vi "GCM_Interface.vi"() -> ()   [LabVIEW 2014]
uses:
  <vilib>/Utility/miscctls.llb/LVPointTypeDef.ctl
  Utilites/Controls/GCM_Data.ctl
  Framework/_Plugins/GCMPlugin/GCMPlugin.lvclass
  Framework/_Plugins/_EmptyPlugin/_EmptyPlugin.lvclass
  Framework/SelectedPluginStorage/SelectedPluginStorage.lvclass
  Framework/_Plugins/GCMSettingsScreen/GCMSettingsScreen.lvclass
  Utilites/Controls/GCM_State.ctl
  Framework/_Plugins/_LVCMPlugin/GCMPlugin_EventsOut.ctl
  Framework/_Plugins/GCMPlugin/GCMPlugin.lvclass/GCMPlugin.ctl
  <vilib>/Utility/cursorutil.llb/Set Cursor (Icon Pict).vi
  Framework/PluginsThread/PluginsLoaderService/PluginsLoaderService.lvclass
  Framework/PluginsThread/PluginsLoaderCommander/PluginsLoaderCommander.lvclass
panel:
  in  "SettingsButton":bool
  out "Item Type":string="Item type"
  out "Current Item":string="Item name"
  in  "Stay on top?":bool
  in  "Plugins":i32(listbox)
  in  "VeritechLogo":bool
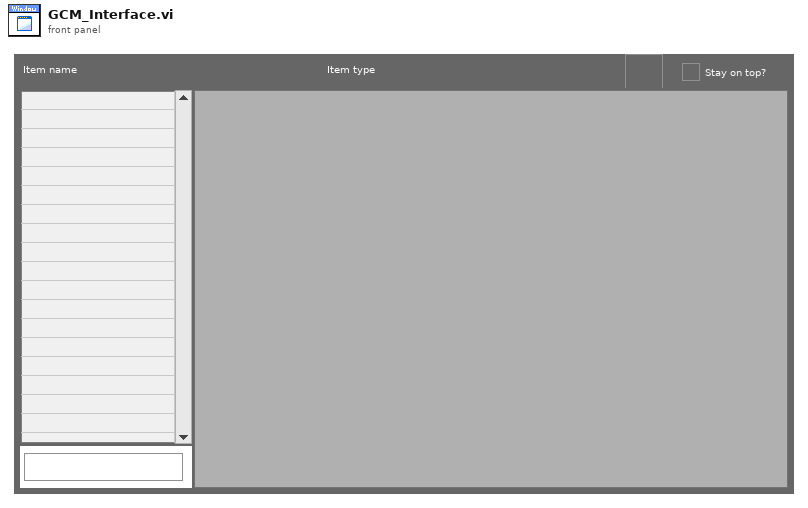
[diagram p1: front panel]
types:
  T1 = typedef "LVPointTypeDef.ctl" = cluster{"Horizontal":i16, "Vertical":i16}
  T2 = typedef "GCMPlugin.lvclass/GCMPlugin_EventsOut.ctl" = cluster{"ItemEdited":refnum<user-event>}
  T3 = typedef "GCM_State.ctl" = enum16{"Initialize", "WaitForEvent", "ShowPluginInterface", "Stop", "LoadDefaultPlugin"}
  T4 = typedef "GCM_Data.ctl" = cluster{"CurrentProjectItem":refnum<vi>, "AvailablePlugins":refnum<class "GCMPlugin.lvclass">[], "EmptyPlugin":refnum<class "_EmptyPlugin.lvclass">, "CurrentPlugin":refnum<class "GCMPlugin.lvclass">, "SelectedPluginStorage":refnum<class "SelectedPluginStorage.lvclass">, "SettingsPlugin":refnum<class "GCMSettingsScreen.lvclass">}
  T5 = enum32{"Invalid", "Default", "Floating", "Floating/Auto-Hide", "Modal"}
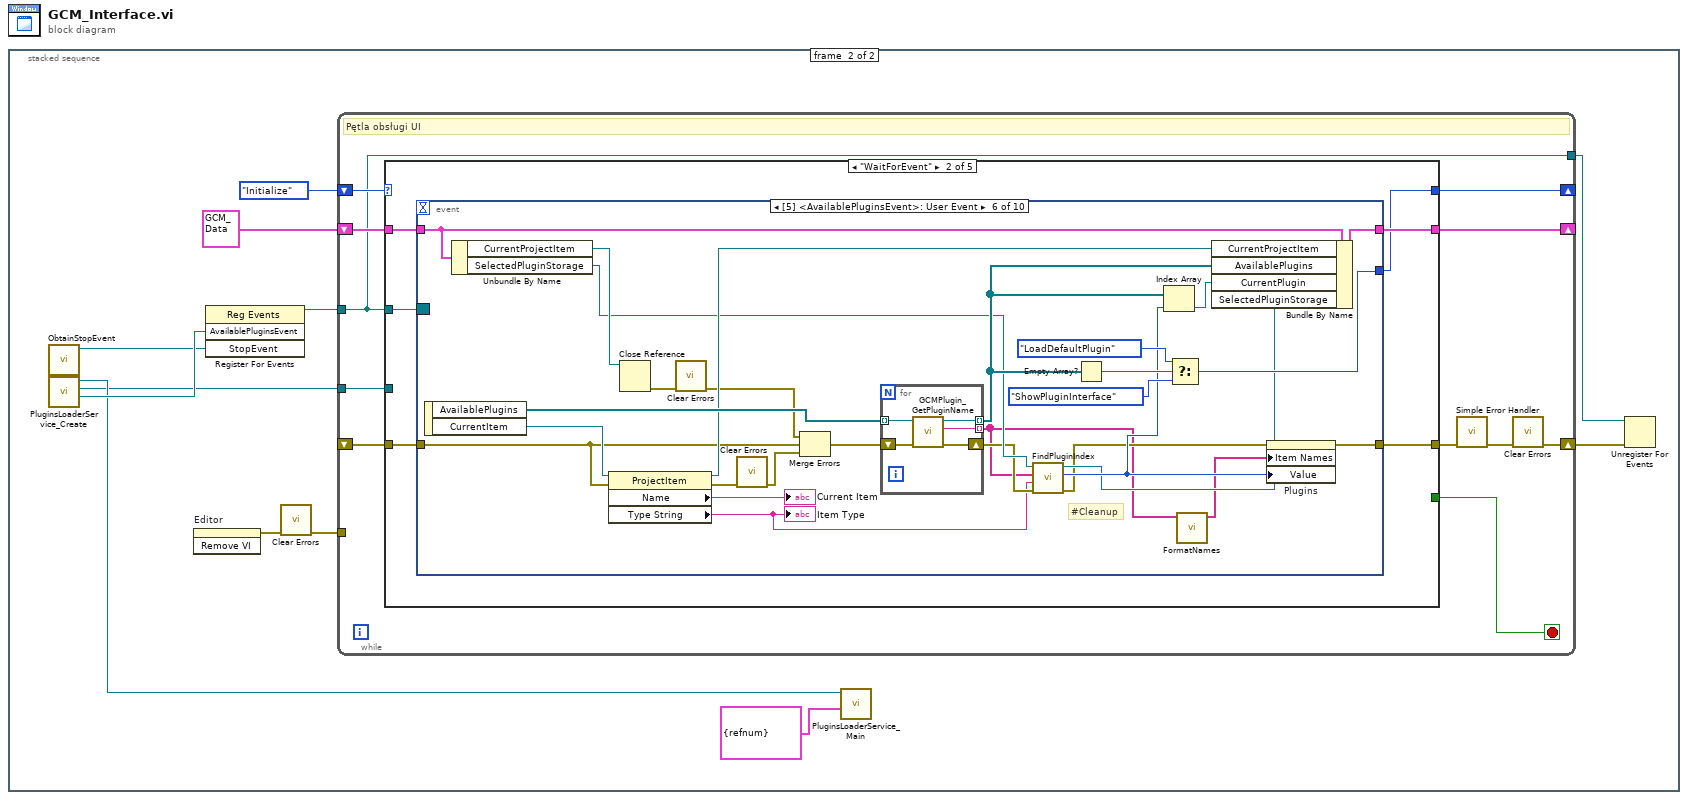
[diagram p0: block diagram]
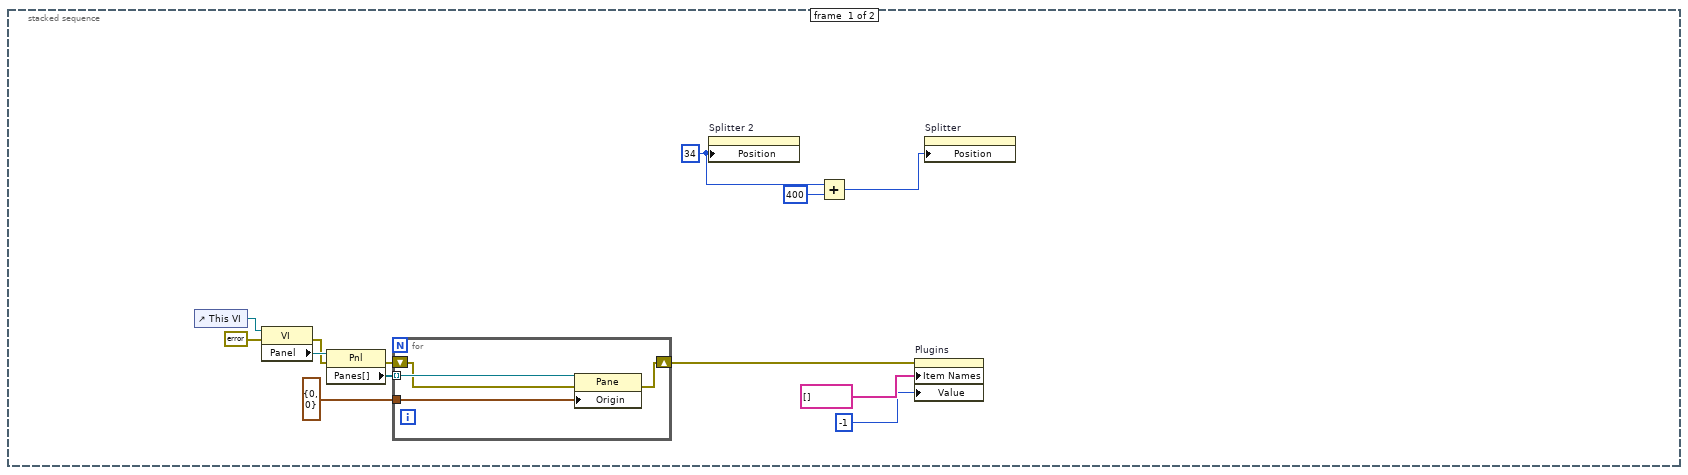
[diagram p2: hidden frame]
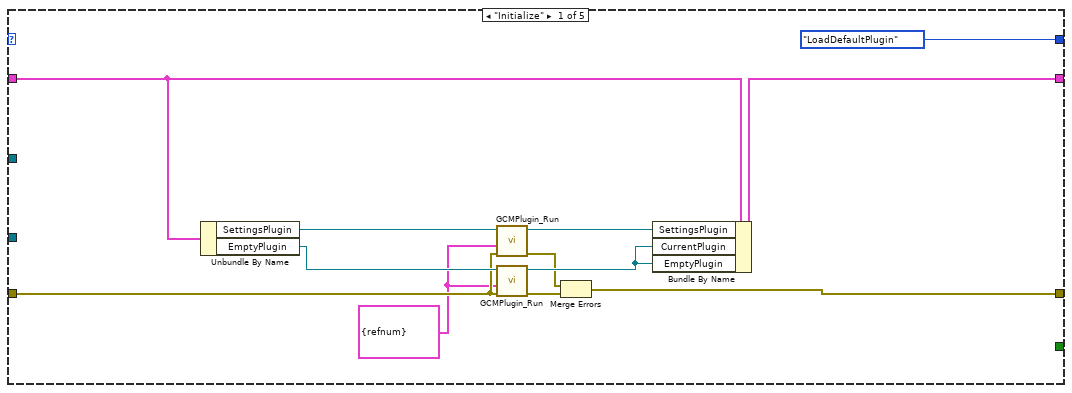
[diagram p3: hidden frame]
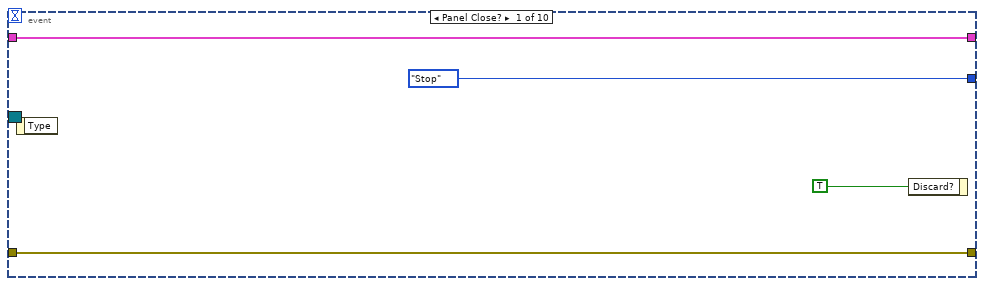
[diagram p4: hidden frame]
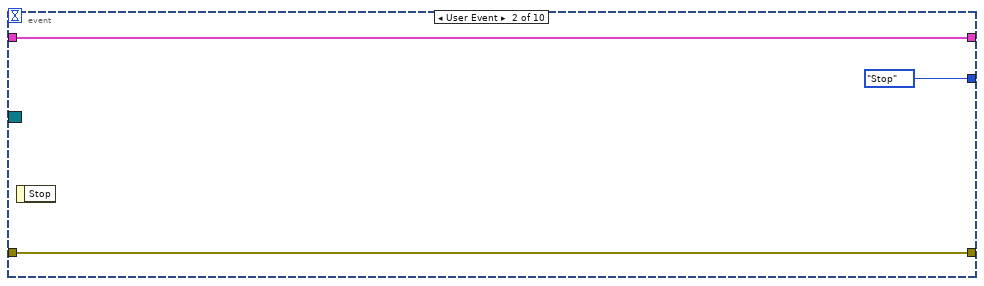
[diagram p5: hidden frame]
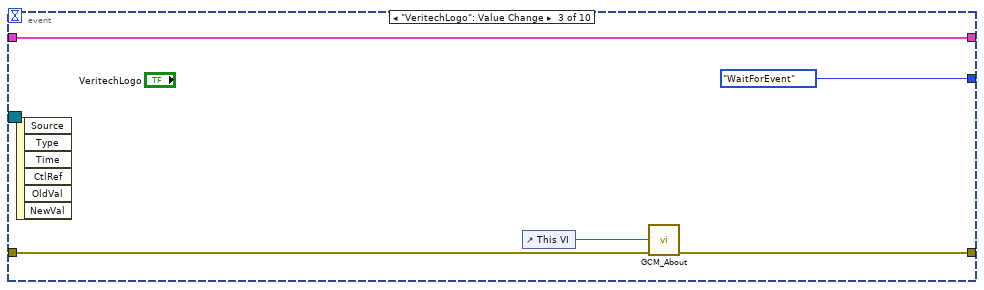
[diagram p6: hidden frame]
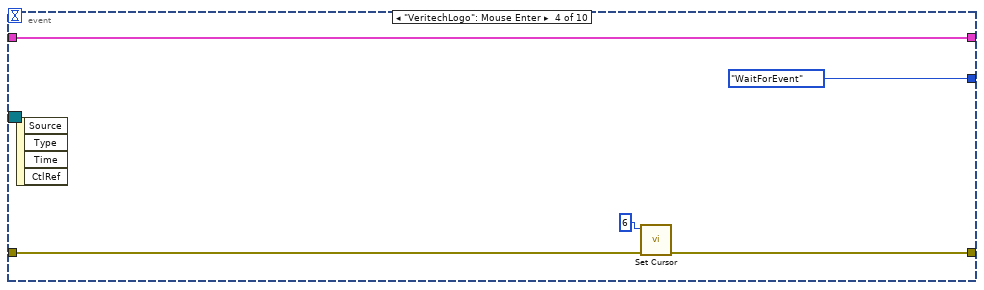
[diagram p7: hidden frame]
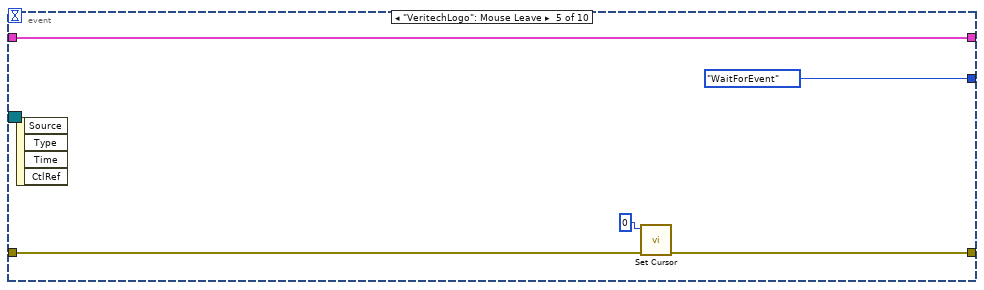
[diagram p8: hidden frame]
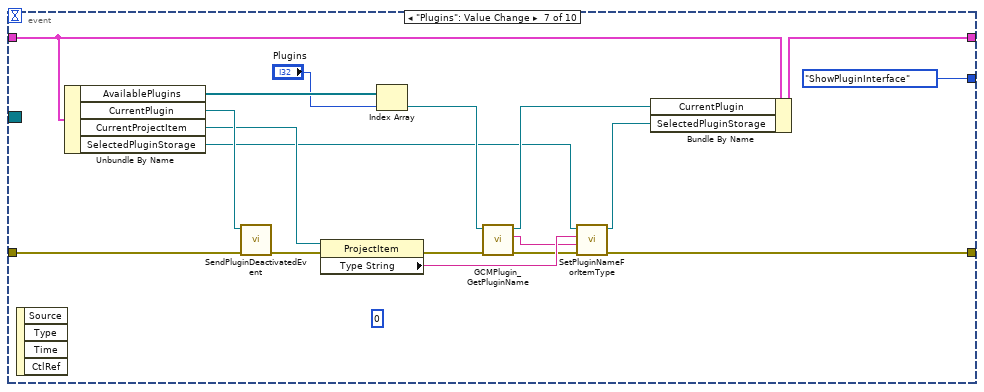
[diagram p9: hidden frame]
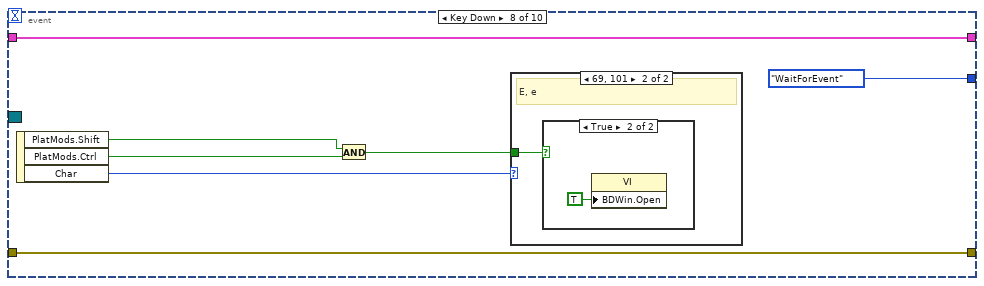
[diagram p10: hidden frame]
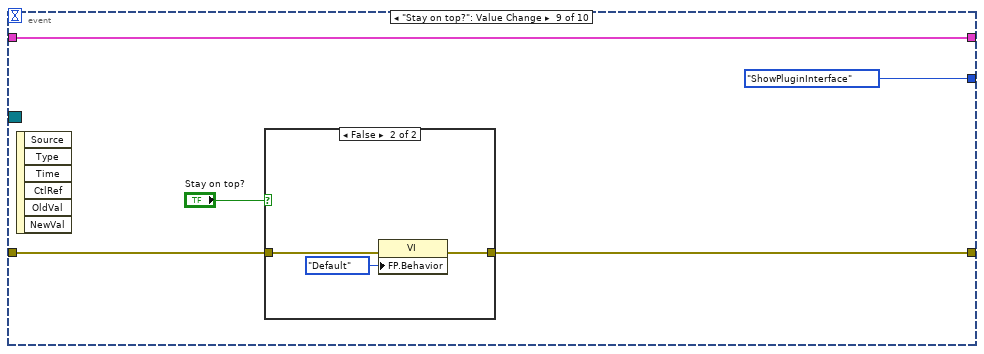
[diagram p13: hidden frame]
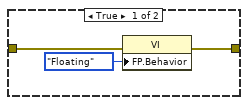
[diagram p14: hidden frame]
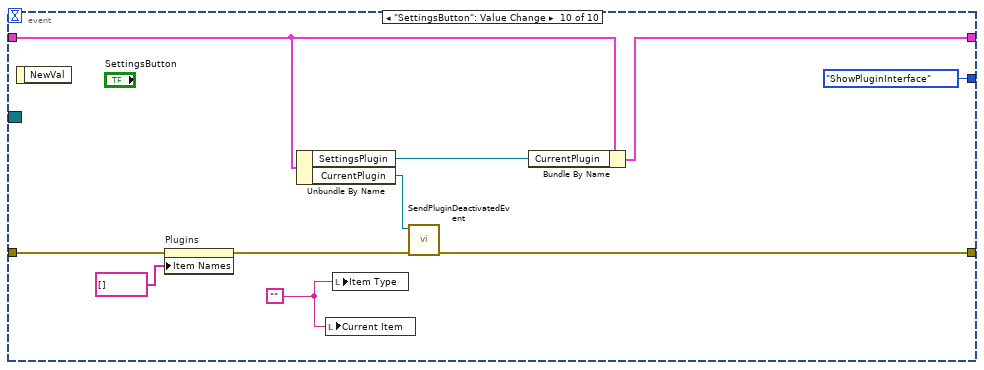
[diagram p15: hidden frame]
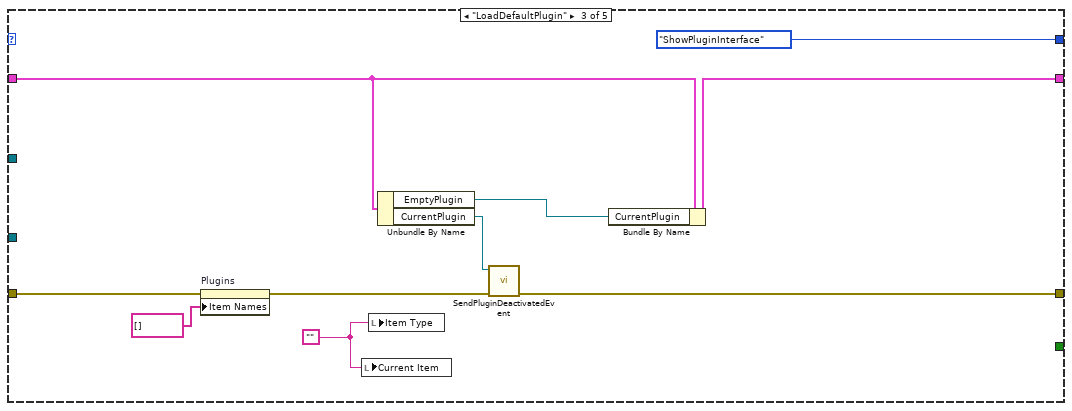
[diagram p16: hidden frame]
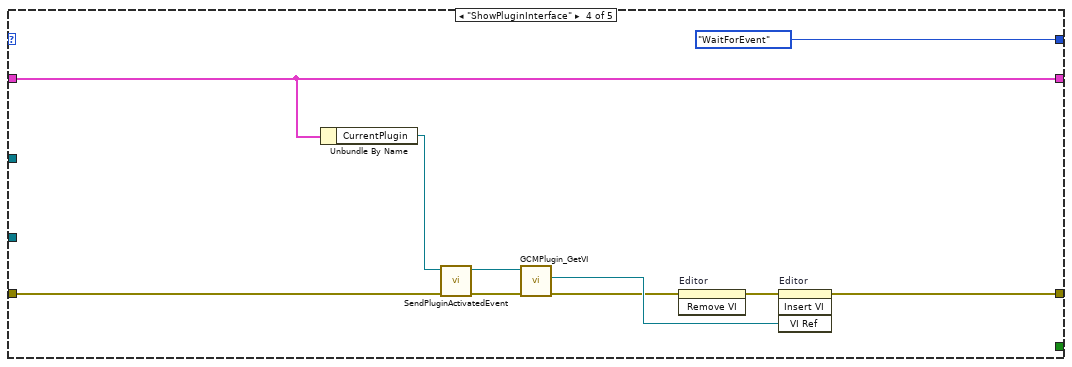
[diagram p17: hidden frame]
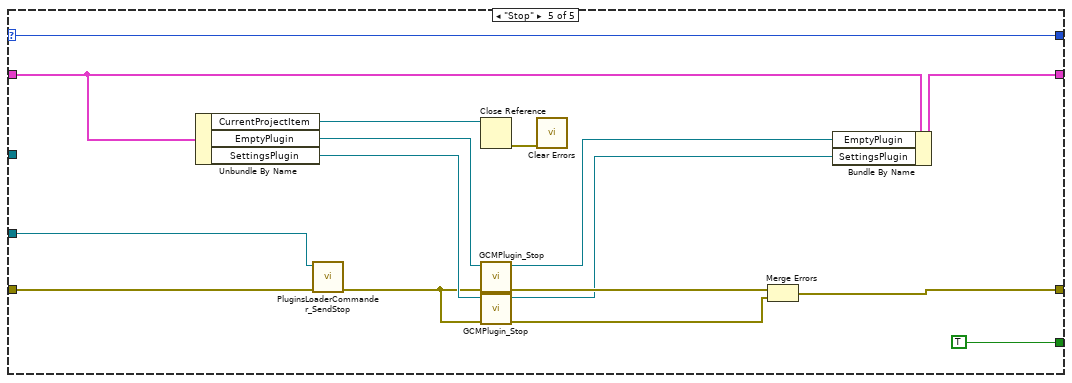
[diagram p18: hidden frame]
diagram:
  n1 = stacked-sequence {
    frame #0 {
      w3 = 34 ("Splitter Position")
      n2 = control-ref of="This VI"() -> (w13:refnum<vi>)
      n3 = property class="VI"(reference=w13, error in=errorcluster {"status"=FALSE, "code"=0, "source"=""} ("error in (no error)")) -> (error out=w11:errorcluster, "Panel"=w12:refnum<vi>)  [unwired: 1 out]
      n4 = property class="Pnl"(reference=w12, error in=w11) -> (error out=w8:errorcluster, "Panes[]"=w9:refnum<vi>[])  [unwired: 1 out]
      n5 = for {
        tunnel: w9 -> [w17] mode=indexing
        shift-right: [w15] -> w6
        shift-left: w8 -> [w16]
        tunnel: T1 {"Horizontal"=0, "Vertical"=0} ("Origin") -> [w14]
        n6 = property class="Pane"(reference=w17, error in=w16, "Origin"=w14) -> (error out=w15:errorcluster)  [unwired: 1 out]
      }
      n7 = property on="Splitter 2" class="Splitter"("Position"=w3) -> ()  [unwired: 2 in, 2 out]
      n8 = Add(x=w3, y=400) -> (x+y=w1:i32)
      n9 = property on="Plugins" class="LstBox (strict)"(error in=w6, "Item Names"=string[] [], "Value"=-1 ("Plugins")) -> ()  [unwired: 1 in, 2 out]
      n10 = property on="Splitter" class="Splitter"("Position"=w1) -> ()  [unwired: 2 in, 2 out]
    }
    frame #1 {
      n11 = call "ObtainStopEvent.vi"() -> ("StopEvent"=w18:refnum<user-event>)  [unwired: 11 in]
      n12 = call "PluginsLoaderService_Create.vi"() -> ("AvailablePluginsEvent"=w26:refnum<user-event>, "Commander"=w19:refnum<class "PluginsLoaderCommander.lvclass">, "PluginsLoaderService out"=w22:refnum<class "PluginsLoaderService.lvclass">)  [unwired: 8 in, 1 out]
      n13 = invoke on="Editor" class="SubPanel" method="Remove VI"() -> (error out=w25:errorcluster)  [unwired: 3 in, 2 out]
      n14 = register-events(w26, w18) -> (reference out=w27:refnum<event-registration>)  [unwired: 2 in, 1 out]
      n15 = call <vilib>:"Clear Errors.vi"("error in (no error)"=w25) -> ("error out"=w20:errorcluster)  [unwired: 5 in, 1 out]
      n16 = while {
        shift-right: [w35] -> w29
        shift-left: _ -> [w40]
        shift-right: [w38] -> _
        shift-left: T4 {"CurrentProjectItem"=refnum, "AvailablePlugins"=[], "EmptyPlugin"=refnum, "CurrentPlugin"=refnum, "SelectedPluginStorage"=refnum, "SettingsPlugin"=refnum} ("LVCMData") -> [w39]
        shift-right: [w32] -> _
        shift-left: GCM_State."Initialize" ("f") -> [w33]
        tunnel: w27 -> [w31]
        tunnel: [w31] -> w23
        tunnel: w20 -> [_]
        tunnel: w19 -> [w30]
        stop <- w34 stop-if-true
        # "Pętla obsługi UI"
        n17 = case shown="\"WaitForEvent\"" w33 {
          selector: w33 -> [_ _ _ _ w195]
          tunnel: w31 -> [_ w58 _ _ _]
          tunnel: w40 -> [w42 w57 w169 w172 w197]
          tunnel: w39 -> [w51 w56 w170 w179 w193]
          tunnel: [w50 w55 w166 w179 w188] -> w38
          tunnel: [w44 w54 w163 w178 w184] -> w36
          tunnel: [_ _ _ _ TRUE] -> w34
          tunnel: [GCM_State."LoadDefaultPlugin" ("f") w53 GCM_State."ShowPluginInterface" ("f") GCM_State."WaitForEvent" ("f") w195] -> w32
          tunnel: w30 -> [_ _ _ _ w194]
          frame "Initialize" {
            w41 = T2 {"ItemEdited"=refnum} ("EventsOut")
            n18 = Unbundle By Name(w51) -> ("SettingsPlugin"=w49:refnum<class "GCMSettingsScreen.lvclass">, "EmptyPlugin"=w47:refnum<class "_EmptyPlugin.lvclass">)
            n19 = call "GCMPlugin_Run.vi"("error in (no error)"=w42, "EventsOut"=w41, "_LVCMPlugin in"=w49) -> ("error out"=w43:errorcluster, "_LVCMPlugin out"=w48:refnum<class "GCMSettingsScreen.lvclass">)  [unwired: 7 in]
            n20 = call "GCMPlugin_Run.vi"("error in (no error)"=w42, "EventsOut"=w41, "_LVCMPlugin in"=w47) -> ("error out"=w45:errorcluster, "_LVCMPlugin out"=w46:refnum<class "_EmptyPlugin.lvclass">)  [unwired: 7 in]
            n21 = Merge Errors(w43, w45) -> (w44:errorcluster)
            n22 = Bundle By Name(cluster=w51, "SettingsPlugin"=w48, "CurrentPlugin"=w46, "EmptyPlugin"=w46) -> (w50:T4)
          }
          frame "WaitForEvent" {
            n23 = event shown="[5] <AvailablePluginsEvent>: User Event" {
              selector: w58 -> [_ _ _ _ _ _ _ _ _ _]
              dyn-events: _ -> [_ _ _ _ _ _ _ _ _ _]
              timeout: _ -> [_ _ _ _ _ _ _ _ _ _]
              tunnel: w57 -> [w62 w65 w69 w73 w78 w99 w131 w138 w145 w153]
              tunnel: [w62 w65 w68 w72 w77 w107 w117 w138 w143 w157] -> w54
              tunnel: w56 -> [w61 w64 w70 w75 w80 w97 w128 w135 w144 w159]
              tunnel: [w61 w64 w70 w75 w80 w106 w126 w135 w144 w158] -> w55
              tunnel: [GCM_State."Stop" ("LVCMState") GCM_State."Stop" ("f") GCM_State."WaitForEvent" ("f") GCM_State."WaitForEvent" ("f") GCM_State."WaitForEvent" ("f") w102 GCM_State."ShowPluginInterface" ("f") GCM_State."WaitForEvent" ("f") GCM_State."ShowPluginInterface" ("f") GCM_State."ShowPluginInterface" ("f")] -> w53
              event Panel Close? {
                n24 = event-data() -> ()  [unwired: 1 in, 1 out]
                n25 = event-data("Discard?"=TRUE) -> ()  [unwired: 1 in, 1 out]
              }
              event User Event {
                n26 = event-data() -> ()  [unwired: 1 in, 1 out]
              }
              event "VeritechLogo": Value Change {
                n27 = event-data() -> ()  [unwired: 1 in, 6 out]
                n28 = control-ref of="This VI"() -> (w67:refnum<vi>)
                n29 = call "GCM_About.vi"("error in"=w69, "VI reference"=w67) -> ("error out"=w68:errorcluster)  [unwired: 9 in]
              }
              event "VeritechLogo": Mouse Enter {
                n30 = event-data() -> ()  [unwired: 1 in, 4 out]
                n31 = call-poly <vilib>:"Set Cursor.vi"("error in (no error)"=w73, "icon"=u16 6) -> ("error out"=w72:errorcluster)  [unwired: 8 in, 1 out]
              }
              event "VeritechLogo": Mouse Leave {
                n32 = event-data() -> ()  [unwired: 1 in, 4 out]
                n33 = call-poly <vilib>:"Set Cursor.vi"("error in (no error)"=w78, "icon"=u16 0) -> ("error out"=w77:errorcluster)  [unwired: 8 in, 1 out]
              }
              event User Event {
                # "#Cleanup"
                n34 = event-data() -> ("AvailablePlugins"=w108:refnum<class "GCMPlugin.lvclass">[], "CurrentItem"=w101:refnum<vi>)  [unwired: 1 in]
                n35 = Unbundle By Name(w97) -> ("CurrentProjectItem"=w96:refnum<vi>, "SelectedPluginStorage"=w88:refnum<class "SelectedPluginStorage.lvclass">)
                n36 = property class="ProjectItem"(reference=w101, error in=w99) -> (reference out=w100:refnum<vi>, error out=w98:errorcluster, "Name"=→"Current Item":string, "Type String"=w81:string)
                "Item Type" <- w81
                n37 = Close Reference(reference=w96) -> (error out=w93:errorcluster)  [unwired: 1 in]
                n38 = call <vilib>:"Clear Errors.vi"("error in (no error)"=w93) -> ("error out"=w92:errorcluster)  [unwired: 5 in, 1 out]
                n39 = call <vilib>:"Clear Errors.vi"("error in (no error)"=w98) -> ("error out"=w94:errorcluster)  [unwired: 5 in, 1 out]
                n40 = Merge Errors(w92, w99, w94) -> (w95:errorcluster)
                n41 = for {
                  tunnel: [w112] -> w84 mode=indexing
                  shift-right: [w111] -> w86
                  shift-left: w95 -> [w113]
                  tunnel: [w110] -> w91 mode=indexing
                  tunnel: w108 -> [w109] mode=indexing
                  n42 = call-dynamic "GCMPlugin_GetPluginName.vi"("error in (no error)"=w113, "_LVCMPlugin in"=w109) -> ("error out"=w111:errorcluster, "PluginName"=w112:string, "_LVCMPlugin out"=w110:refnum<class "GCMPlugin.lvclass">)  [unwired: 7 in]
                }
                n43 = call "FindPluginIndex.vi"("error in (no error)"=w86, "ItemType"=w81, "AvailablePluginsNames"=w84, "SelectedPluginStorage in"=w88) -> ("error out"=w85:errorcluster, "PluginIndex"=w89:i32, "SelectedPluginStorage out"=w87:refnum<class "SelectedPluginStorage.lvclass">)  [unwired: 5 in]
                n44 = Empty Array?(array=w91) -> (empty?=w105:bool)
                n45 = Index Array(array=w91, index=w89) -> (element=w90:refnum<class "GCMPlugin.lvclass">)
                n46 = Select(t=GCM_State."LoadDefaultPlugin" ("f"), s=w105, f=GCM_State."ShowPluginInterface") -> (s? t:f=w102:T3)
                n47 = call "FormatNames.vi"("Names"=w84) -> ("Names out"=w83:string[])  [unwired: 10 in]
                n48 = Bundle By Name(cluster=w97, "CurrentProjectItem"=w100, "AvailablePlugins"=w91, "CurrentPlugin"=w90, "SelectedPluginStorage"=w87) -> (w106:T4)
                n49 = property on="Plugins" class="LstBox (strict)"(error in=w85, "Item Names"=w83, "Value"=w89) -> (error out=w107:errorcluster)  [unwired: 1 in, 1 out]
              }
              event "Plugins": Value Change {
                (unwired) 0 ("Plugins")
                n50 = event-data() -> ()  [unwired: 1 in, 4 out]
                n51 = Unbundle By Name(w128) -> ("AvailablePlugins"=w129:refnum<class "GCMPlugin.lvclass">[], "CurrentPlugin"=w127:refnum<class "GCMPlugin.lvclass">, "CurrentProjectItem"=w125:refnum<vi>, "SelectedPluginStorage"=w115:refnum<class "SelectedPluginStorage.lvclass">)
                n52 = call "SendPluginDeactivatedEvent.vi"("error in (no error)"=w131, "_LVCMPlugin in"=w127) -> ("error out"=w124:errorcluster)  [unwired: 8 in, 1 out]
                n53 = property class="ProjectItem"(reference=w125, error in=w124) -> (error out=w123:errorcluster, "Type String"=w122:string)  [unwired: 1 out]
                n54 = Index Array(array=w129, index="Plugins") -> (element=w120:refnum<class "GCMPlugin.lvclass">)
                n55 = call-dynamic "GCMPlugin_GetPluginName.vi"("error in (no error)"=w123, "_LVCMPlugin in"=w120) -> ("error out"=w121:errorcluster, "PluginName"=w118:string, "_LVCMPlugin out"=w119:refnum<class "GCMPlugin.lvclass">)  [unwired: 7 in]
                n56 = call "SetPluginNameForItemType.vi"("error in (no error)"=w121, "PluginName"=w118, "ItemType"=w122, "SelectedPluginStorage in"=w115) -> ("error out"=w117:errorcluster, "SelectedPluginStorage out"=w116:refnum<class "SelectedPluginStorage.lvclass">)  [unwired: 6 in]
                n57 = Bundle By Name(cluster=w128, "CurrentPlugin"=w119, "SelectedPluginStorage"=w116) -> (w126:T4)
              }
              event Key Down {
                n58 = event-data() -> ("PlatMods.Shift"=w132:bool, "PlatMods.Ctrl"=w136:bool, "Char"=w137:i16)  [unwired: 1 in]
                n59 = And(x=w132, y=w136) -> (x .and. y?=w133:bool)
                n60 = case shown="69, 101" w137 {
                  tunnel: w133 -> [_ w139]
                  frame Default {
                  }
                  frame 69, 101 {
                    # "E, e"
                    n61 = case shown="True" w139 {
                      frame False {
                      }
                      frame True {
                        n62 = property class="VI"("BDWin.Open"=TRUE ("Block Diagram Window:Open")) -> ()  [unwired: 2 in, 2 out]
                      }
                    }
                  }
                }
              }
              event "Stay on top?": Value Change {
                n63 = event-data() -> ()  [unwired: 1 in, 6 out]
                n64 = case shown="False" "Stay on top?" {
                  tunnel: w145 -> [w148 w151]
                  tunnel: [w147 w150] -> w143
                  frame True {
                    n65 = property class="VI"(error in=w148, "FP.Behavior"=T5."Floating" ("Front Panel Window:Behavior")) -> (error out=w147:errorcluster)  [unwired: 1 in, 1 out]
                  }
                  frame False {
                    n66 = property class="VI"(error in=w151, "FP.Behavior"=T5."Default" ("Front Panel Window:Behavior")) -> (error out=w150:errorcluster)  [unwired: 1 in, 1 out]
                  }
                }
              }
              event "SettingsButton": Value Change {
                w154 = ""
                n67 = event-data() -> ()  [unwired: 1 in, 1 out]
                n68 = property on="Plugins" class="LstBox (strict)"(error in=w153, "Item Names"=string[] []) -> (error out=w152:errorcluster)  [unwired: 1 in, 1 out]
                n69 = Unbundle By Name(w159) -> ("SettingsPlugin"=w160:refnum<class "GCMSettingsScreen.lvclass">, "CurrentPlugin"=w161:refnum<class "GCMPlugin.lvclass">)
                n70 = local write "Current Item"(w154) -> ()
                n71 = local write "Item Type"(w154) -> ()
                n72 = call "SendPluginDeactivatedEvent.vi"("error in (no error)"=w152, "_LVCMPlugin in"=w161) -> ("error out"=w157:errorcluster)  [unwired: 8 in, 1 out]
                n73 = Bundle By Name(cluster=w159, "CurrentPlugin"=w160) -> (w158:T4)
              }
            }
          }
          frame "LoadDefaultPlugin" {
            w162 = ""
            n74 = property on="Plugins" class="LstBox (strict)"(error in=w169, "Item Names"=string[] []) -> (error out=w168:errorcluster)  [unwired: 1 in, 1 out]
            n75 = local write "Current Item"(w162) -> ()
            n76 = local write "Item Type"(w162) -> ()
            n77 = Unbundle By Name(w170) -> ("EmptyPlugin"=w164:refnum<class "_EmptyPlugin.lvclass">, "CurrentPlugin"=w165:refnum<class "GCMPlugin.lvclass">)
            n78 = call "SendPluginDeactivatedEvent.vi"("error in (no error)"=w168, "_LVCMPlugin in"=w165) -> ("error out"=w163:errorcluster)  [unwired: 8 in, 1 out]
            n79 = Bundle By Name(cluster=w170, "CurrentPlugin"=w164) -> (w166:T4)
          }
          frame "ShowPluginInterface" {
            n80 = Unbundle By Name(w179) -> ("CurrentPlugin"=w175:refnum<class "GCMPlugin.lvclass">)
            n81 = call "SendPluginActivatedEvent.vi"("error in (no error)"=w172, "_LVCMPlugin in"=w175) -> ("error out"=w173:errorcluster, "_LVCMPlugin out"=w174:refnum<class "GCMPlugin.lvclass">)  [unwired: 8 in]
            n82 = call "GCMPlugin_GetVI.vi"("error in (no error)"=w173, "_LVCMPlugin in"=w174) -> ("error out"=w176:errorcluster, "VI"=w177:refnum<vi>)  [unwired: 7 in, 1 out]
            n83 = invoke on="Editor" class="SubPanel" method="Remove VI"(error in=w176) -> (error out=w180:errorcluster)  [unwired: 2 in, 2 out]
            n84 = invoke on="Editor" class="SubPanel" method="Insert VI"(error in=w180, "VI Ref"=w177) -> (error out=w178:errorcluster)  [unwired: 2 in, 3 out]
          }
          frame "Stop" {
            n85 = Unbundle By Name(w193) -> ("CurrentProjectItem"=w192:refnum<vi>, "EmptyPlugin"=w189:refnum<class "_EmptyPlugin.lvclass">, "SettingsPlugin"=w186:refnum<class "GCMSettingsScreen.lvclass">)
            n86 = call "PluginsLoaderCommander_SendStop.vi"("error in (no error)"=w197, "PluginsLoaderCommander in"=w194) -> ("error out"=w182:errorcluster)  [unwired: 8 in, 1 out]
            n87 = Close Reference(reference=w192) -> (error out=w191:errorcluster)  [unwired: 1 in]
            n88 = call "GCMPlugin_Stop.vi"("error in (no error)"=w182, "_LVCMPlugin in"=w189) -> ("error out"=w190:errorcluster, "_LVCMPlugin out"=w187:refnum<class "_EmptyPlugin.lvclass">)  [unwired: 8 in]
            n89 = call "GCMPlugin_Stop.vi"("error in (no error)"=w182, "_LVCMPlugin in"=w186) -> ("error out"=w183:errorcluster, "_LVCMPlugin out"=w185:refnum<class "GCMSettingsScreen.lvclass">)  [unwired: 8 in]
            n90 = call <vilib>:"Clear Errors.vi"("error in (no error)"=w191) -> ()  [unwired: 5 in, 2 out]
            n91 = Merge Errors(w190, w183) -> (w184:errorcluster)
            n92 = Bundle By Name(cluster=w193, "EmptyPlugin"=w187, "SettingsPlugin"=w185) -> (w188:T4)
          }
        }
        n93 = call <vilib>:"Simple Error Handler.vi"("error in (no error)"=w36) -> ("error out"=w37:errorcluster)  [unwired: 4 in, 4 out]
        n94 = call <vilib>:"Clear Errors.vi"("error in (no error)"=w37) -> ("error out"=w35:errorcluster)  [unwired: 5 in, 1 out]
      }
      n95 = call "PluginsLoaderService_Main.vi"("EventsOut"=T2 {"ItemEdited"=refnum}, "PluginsLoaderService"=w22) -> ()  [unwired: 10 in]
      n96 = Unregister For Events(event registration refnum=w23, error in=w29) -> ()  [unwired: 1 out]
    }
  }
